vi "Read States.vi"(8 "error in (no error)":errorcluster, 11 "TestTactic in":refnum<class "TestTactic.lvclass">) -> (0 "error out":errorcluster, 2 "Enum":T1, 3 "TestTactic out":refnum<class "TestTactic.lvclass">)   [LabVIEW 2023, in "TestTactic.lvclass"]
uses:
  TestTactic.lvclass
  STP_Parameters/TestSkills.ctl
  TestTactic.lvclass/TestTactic.ctl
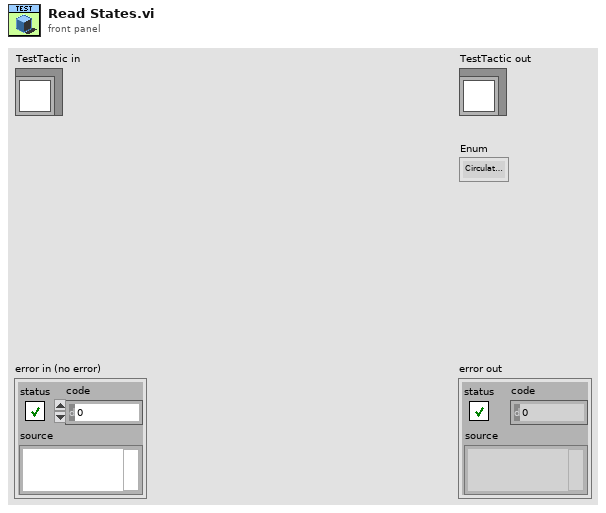
[diagram p1: front panel]
types:
  T1 = typedef "TestSkills.ctl" = enum16{"CirculateBall", "ProtectBall", "ReceivePass", "GoTo"}
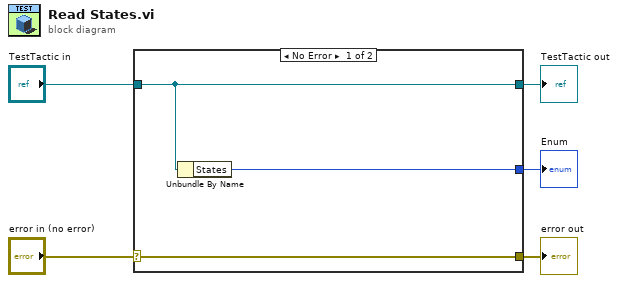
[diagram p0: block diagram]
diagram:
  n1 = case shown="No Error" "error in (no error)" {
    selector: "error in (no error)" -> [w8 w9]
    tunnel: [w8 w9] -> w4
    tunnel: [w7 w10] -> w2
    tunnel: "TestTactic in" -> [w7 w10]
    tunnel: [w6 _] -> w1
    frame No Error {
      n2 = Unbundle By Name(w7) -> ("States"=w6:T1)
    }
    frame Error {
    }
  }
  "error out" <- w4
  "TestTactic out" <- w2
  "Enum" <- w1
